vi "HeaderAction.vi"(0 "InstrClass":refnum<class "MultiHarp150.lvclass"> caption="DNL_LabVIEW Object in", 11 "error in (no error)":errorcluster caption="entrée d'erreur (pas d'erreur)") -> (4 "InstrClassOut":refnum<class "MultiHarp150.lvclass"> caption="DNL_LabVIEW Object out", 6 "DataNames":string[](array[string]), 8 "Instr Name":string, 10 "HeaderString":string, 13 "ArrDisplayNames":string[](array[string]), 14 "DisplayNames":string[](array[string]), 15 "error out":errorcluster caption="sortie d'erreur")   [LabVIEW 2019, in "MultiHarp150.lvclass"]
uses:
  MultiHarp150.lvclass
  C:/Programmes Labview/LabScanV1A/DevicesClass/BaseDevice/BaseDevice.lvclass
  <userlib>/MultiHarp150/MH_MeasMode.ctl
  <userlib>/MultiHarp150/MH_RefSource.ctl
  MultiHarp150.lvclass/MultiHarp150.ctl
  BaseDevice/BaseDevice.lvclass/BaseDevice.ctl
  BaseDevice/Accessor/GetBaseDataPath.vi
  BaseDevice/BaseDevice.lvclass
panel:
  out "refsource":T1
  out "Mode":T2 items=["HIST"=0, "T2"=2, "T3"=3]
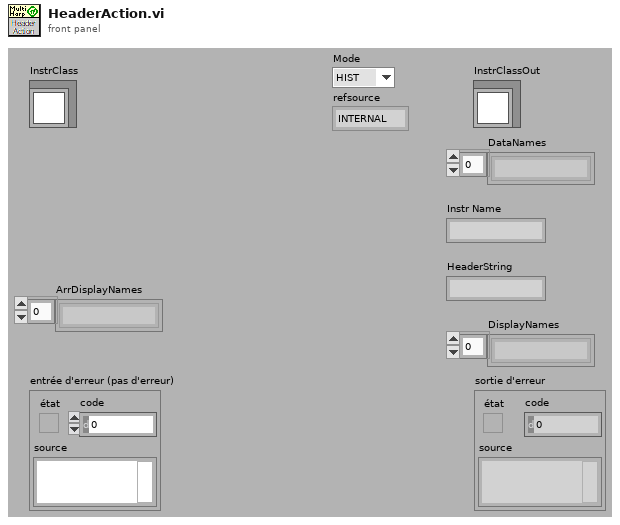
[diagram p1: front panel]
types:
  T1 = typedef "MH_RefSource.ctl" = enum16{"INTERNAL", "EXTERNAL_10MHZ", "WR_MASTER_GENERIC", "WR_SLAVE_GENERIC", "WR_GRANDM_GENERIC", "EXTN_GPS_PPS", "EXTN_GPS_PPS_UART", "WR_MASTER_MHARP", "WR_SLAVE_MHARP", "WR_GRANDM_MHARP"}
  T2 = typedef "MH_MeasMode.ctl" = i32
  T3 = typedef "MultiHarp150.lvclass/MultiHarp150_Func.ctl" = enum16{"ReadHistogram (Ph)", "ReadT2 (Ph)", "ReadT3 (Ph)", "ReadCount (Ph)"}
  T4 = typedef "MH_InputChannel_LS.ctl" = cluster{"Name":string, "Enable":bool, "Edge":i32, "Level":i32, "Offset":i32, "UseDeadTime":bool, "DeadTime":i32}
  T5 = cluster{"TagIdent":string, "TagIndex":i32, "TagType":i32, "TagValue":i64, "TagAuxData":string}[]
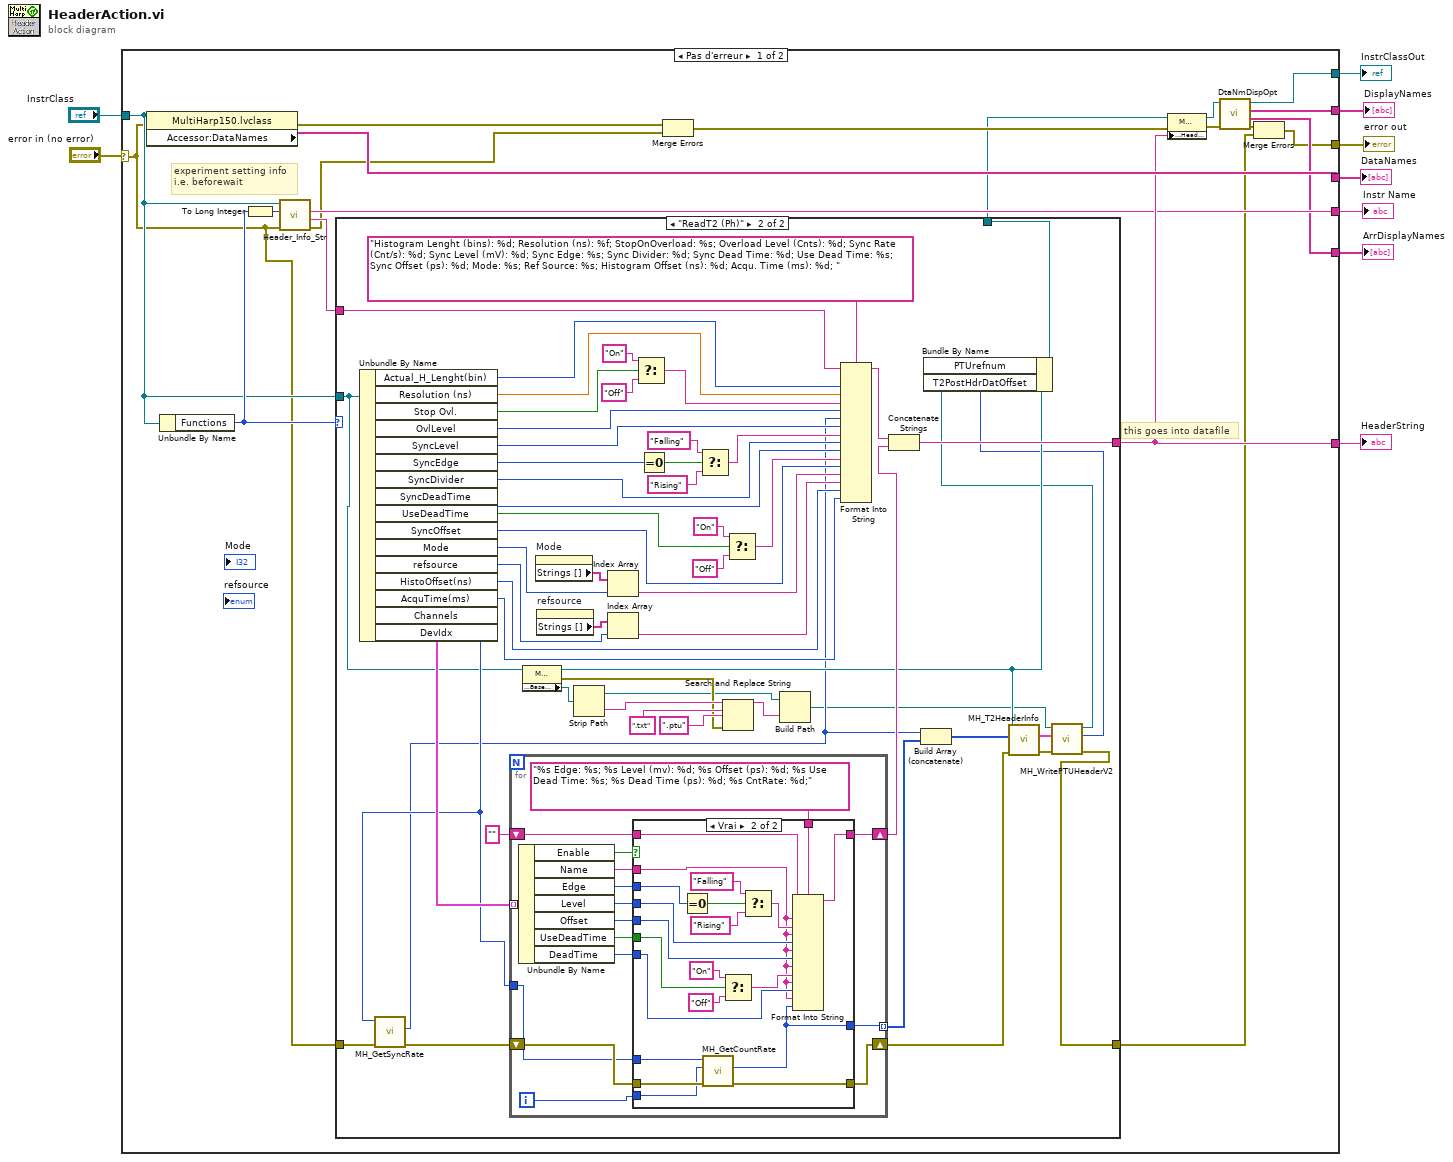
[diagram p0: block diagram]
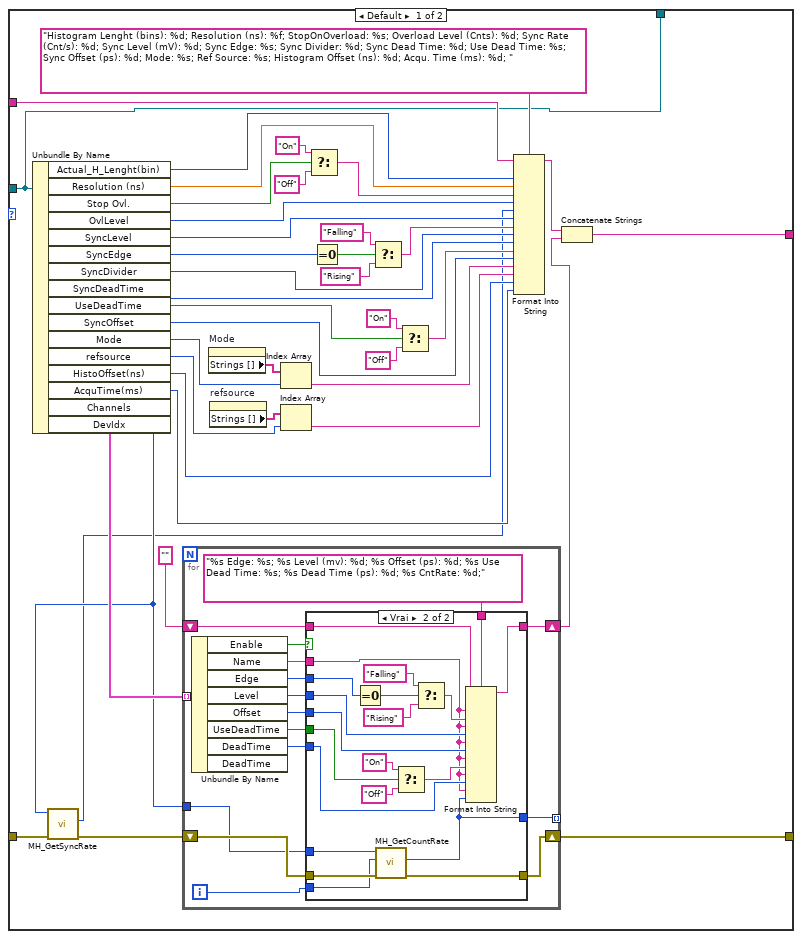
[diagram p2: hidden frame]
diagram:
  n1 = case shown="Pas d'erreur" "error in (no error)" {
    selector: "error in (no error)" -> [w14 w207]
    tunnel: [w27 _] -> w8
    tunnel: [w29 _] -> w7
    tunnel: "InstrClass" -> [w15 w208]
    tunnel: [w12 w207] -> w5
    tunnel: [w24 w208] -> w3
    tunnel: [w21 _] -> w4
    tunnel: [w22 _] -> w2
    tunnel: [w16 _] -> w1
    frame No Error {
      # "this goes into datafile"
      # "experiment setting info\ni.e. beforewait"
      n2 = property class="MultiHarp150.lvclass"(reference=w15, error in=w14) -> (error out=w28:errorcluster, "Accessor:DataNames"=w29:string[])  [unwired: 1 out]
      n3 = Unbundle By Name(w15) -> ("Functions"=w18:T3)
      n4 = To Long Integer(number=w18) -> (32bit integer=w17:i32)
      n5 = call-dynamic "Header_Info_Str.vi"("error in (no error)"=w14, "Functions"=w17, "DefaultDev in"=w15) -> ("error out"=w13:errorcluster, "HdrInfoStr"=w20:string, "InstrumentName"=w21:string)  [unwired: 5 in, 1 out]
      n6 = case shown="\"ReadT2 (Ph)\"" w18 {
        tunnel: [w39 w136] -> w27
        tunnel: w20 -> [w70 w167]
        tunnel: w15 -> [w30 w110]
        tunnel: w14 -> [w38 w135]
        tunnel: [w31 w124] -> w11
        tunnel: [w30 w113] -> w10
        frame Default {
          n7 = Unbundle By Name(w30) -> ("Actual_H_Lenght(bin)"=w48:i32, "Resolution (ns)"=w50:dbl, "Stop Ovl."=w52:bool, "OvlLevel"=w53:u32, "SyncLevel"=w34:i32, "SyncEdge"=w68:i32, "SyncDivider"=w64:i32, "SyncDeadTime"=w63:i32, "UseDeadTime"=w58:bool, "SyncOffset"=w49:i32, "Mode"=w55:T2, "refsource"=w44:T1, "HistoOffset(ns)"=w42:i32, "AcquTime(ms)"=w41:i32, "Channels"=w40:T4[], "DevIdx"=w36:i32)
          n8 = call <userlib>:"MH_GetSyncRate.vi"("error in (no error)"=w38, "devidx"=w36) -> ("error out"=w37:errorcluster, "syncrate"=w33:i32)  [unwired: 7 in, 1 out]
          n9 = for {
            tunnel: w40 -> [w86] mode=indexing
            shift-right: [w76] -> w32
            shift-left: "" -> [w77]
            tunnel: w36 -> [w74]
            shift-right: [w73] -> w31
            shift-left: w37 -> [w75]
            tunnel: [w71] -> _ mode=indexing
            i -> [w72]
            n10 = Unbundle By Name(w86) -> ("Enable"=w78:bool, "Name"=w79:string, "Edge"=w85:i32, "Level"=w82:i32, "Offset"=w81:i32, "UseDeadTime"=w84:bool, "DeadTime"=w80:i32)  [unwired: 1 out]
            n11 = case shown="Vrai" w78 {
              tunnel: w85 -> [_ w104]
              tunnel: w84 -> [_ w103]
              tunnel: "%s Edge: %s; %s Level (mv): %d; %s Offset (ps): %d; %s Use Dead Time: %s; %s Dead Time (ps): %d; %s CntRate: %d;" -> [_ w97]
              tunnel: w82 -> [_ w101]
              tunnel: w81 -> [_ w100]
              tunnel: w80 -> [_ w98]
              tunnel: w79 -> [_ w90]
              tunnel: w77 -> [w88 w96]
              tunnel: [w88 w95] -> w76
              tunnel: w75 -> [w87 w94]
              tunnel: w74 -> [_ w93]
              tunnel: [w87 w92] -> w73
              tunnel: w72 -> [_ w91]
              tunnel: [_ w89] -> w71
              frame False {
              }
              frame True {
                n12 = Equal To 0?(x=w104) -> (x = 0?=w106:bool)
                n13 = call <userlib>:"MH_GetCountRate.vi"("error in (no error)"=w94, "Channel"=w91, "devidx"=w93) -> ("error out"=w92:errorcluster, "rate"=w89:i32)  [unwired: 6 in, 1 out]
                n14 = Select(t="On", s=w103, f="Off") -> (s? t:f=w99:string)
                n15 = Select(t="Falling", s=w106, f="Rising") -> (s? t:f=w102:string)
                n16 = Format Into String(format string=w97, initial string=w96, w90, w102, w90, w101, w90, w100, w90, w99, w90, w98, w90, w89) -> (resulting string=w95:string)  [unwired: 1 in, 1 out]
              }
            }
          }
          n17 = property on="Mode" class="MDér (strict)"() -> ("Strings []"=w56:string[])  [unwired: 2 in, 2 out]
          n18 = property on="refsource" class="Énum (strict)"() -> ("Strings []"=w45:string[])  [unwired: 2 in, 2 out]
          n19 = Index Array(array=w56, index=w55) -> (element=w47:string)
          n20 = Index Array(array=w45, index=w44) -> (element=w43:string)
          n21 = Select(t="On", s=w52, f="Off") -> (s? t:f=w51:string)
          n22 = Equal To 0?(x=w68) -> (x = 0?=w67:bool)
          n23 = Select(t="Falling", s=w67, f="Rising") -> (s? t:f=w35:string)
          n24 = Select(t="On", s=w58, f="Off") -> (s? t:f=w57:string)
          n25 = Format Into String(format string="Histogram Lenght (bins): %d; Resolution (ns): %f; StopOnOverload: %s; Overload Level (Cnts): %d; Sync Rate (Cnt/s): %d; Sync Level (mV): %d; Sync Edge: %s; Sync Divider: %d; Sync Dead Time: %d; Use Dead Time: %s; Sync Offset (ps): %d; Mode: %s; Ref Source: %s; Histogram Offset (ns): %d; Acqu. Time (ms): %d; " ("chaîne de format"), initial string=w70, w48, w50, w51, w53, w33, w34, w35, w64, w63, w57, w49, w47, w43, w42, w41) -> (resulting string=w54:string)  [unwired: 1 in, 1 out]
          n26 = Concatenate Strings(w54, w32) -> (w39:string)
        }
        frame "ReadT2 (Ph)" {
          n27 = Unbundle By Name(w110) -> ("Actual_H_Lenght(bin)"=w145:i32, "Resolution (ns)"=w147:dbl, "Stop Ovl."=w149:bool, "OvlLevel"=w150:u32, "SyncLevel"=w131:i32, "SyncEdge"=w165:i32, "SyncDivider"=w161:i32, "SyncDeadTime"=w160:i32, "UseDeadTime"=w155:bool, "SyncOffset"=w146:i32, "Mode"=w152:T2, "refsource"=w141:T1, "HistoOffset(ns)"=w139:i32, "AcquTime(ms)"=w138:i32, "Channels"=w137:T4[], "DevIdx"=w133:i32)
          n28 = call <userlib>:"MH_GetSyncRate.vi"("error in (no error)"=w135, "devidx"=w133) -> ("error out"=w134:errorcluster, "syncrate"=w122:i32)  [unwired: 7 in, 1 out]
          n29 = for {
            tunnel: w137 -> [w183] mode=indexing
            shift-right: [w173] -> w130
            shift-left: "" -> [w174]
            tunnel: w133 -> [w171]
            shift-right: [w170] -> w127
            shift-left: w134 -> [w172]
            tunnel: [w168] -> w128 mode=indexing
            i -> [w169]
            n30 = Unbundle By Name(w183) -> ("Enable"=w175:bool, "Name"=w176:string, "Edge"=w182:i32, "Level"=w179:i32, "Offset"=w178:i32, "UseDeadTime"=w181:bool, "DeadTime"=w177:i32)
            n31 = case shown="Vrai" w175 {
              tunnel: w182 -> [_ w201]
              tunnel: w181 -> [_ w200]
              tunnel: "%s Edge: %s; %s Level (mv): %d; %s Offset (ps): %d; %s Use Dead Time: %s; %s Dead Time (ps): %d; %s CntRate: %d;" -> [_ w194]
              tunnel: w179 -> [_ w198]
              tunnel: w178 -> [_ w197]
              tunnel: w177 -> [_ w195]
              tunnel: w176 -> [_ w187]
              tunnel: w174 -> [w185 w193]
              tunnel: [w185 w192] -> w173
              tunnel: w172 -> [w184 w191]
              tunnel: w171 -> [_ w190]
              tunnel: [w184 w189] -> w170
              tunnel: w169 -> [_ w188]
              tunnel: [_ w186] -> w168
              frame False {
              }
              frame True {
                n32 = Equal To 0?(x=w201) -> (x = 0?=w203:bool)
                n33 = call <userlib>:"MH_GetCountRate.vi"("error in (no error)"=w191, "Channel"=w188, "devidx"=w190) -> ("error out"=w189:errorcluster, "rate"=w186:i32)  [unwired: 6 in, 1 out]
                n34 = Select(t="On", s=w200, f="Off") -> (s? t:f=w196:string)
                n35 = Select(t="Falling", s=w203, f="Rising") -> (s? t:f=w199:string)
                n36 = Format Into String(format string=w194, initial string=w193, w187, w199, w187, w198, w187, w197, w187, w196, w187, w195, w187, w186) -> (resulting string=w192:string)  [unwired: 1 in, 1 out]
              }
            }
          }
          n37 = property class="MultiHarp150.lvclass"(reference=w110) -> (reference out=w123:refnum<class "MultiHarp150.lvclass">, error out=w117:errorcluster, "Accessor:BaseDataPath"=w121:path)  [unwired: 1 in]
          n38 = property on="Mode" class="MDér (strict)"() -> ("Strings []"=w153:string[])  [unwired: 2 in, 2 out]
          n39 = property on="refsource" class="Énum (strict)"() -> ("Strings []"=w142:string[])  [unwired: 2 in, 2 out]
          n40 = Strip Path(path=w121) -> (stripped path=w116:path, name=w120:string)
          n41 = Index Array(array=w153, index=w152) -> (element=w144:string)
          n42 = Index Array(array=w142, index=w141) -> (element=w140:string)
          n43 = Select(t="On", s=w149, f="Off") -> (s? t:f=w148:string)
          n44 = Equal To 0?(x=w165) -> (x = 0?=w164:bool)
          n45 = Select(t="Falling", s=w164, f="Rising") -> (s? t:f=w132:string)
          n46 = Search and Replace String(input string=w120, search string=".txt" ("expression régulière"), replace string=".ptu" ("expression régulière"), error in=w117) -> (result string=w115:string)  [unwired: 4 in, 3 out]
          n47 = Select(t="On", s=w155, f="Off") -> (s? t:f=w154:string)
          n48 = Build Path(base path=w116, name or relative path=w115) -> (appended path=w114:path)
          n49 = Format Into String(format string="Histogram Lenght (bins): %d; Resolution (ns): %f; StopOnOverload: %s; Overload Level (Cnts): %d; Sync Rate (Cnt/s): %d; Sync Level (mV): %d; Sync Edge: %s; Sync Divider: %d; Sync Dead Time: %d; Use Dead Time: %s; Sync Offset (ps): %d; Mode: %s; Ref Source: %s; Histogram Offset (ns): %d; Acqu. Time (ms): %d; " ("chaîne de format"), initial string=w167, w145, w147, w148, w150, w122, w131, w132, w161, w160, w154, w146, w144, w140, w139, w138) -> (resulting string=w151:string)  [unwired: 1 in, 1 out]
          n50 = Concatenate Strings(w151, w130) -> (w136:string)
          n51 = Build Array (concatenate)(w122, w128) -> (w129:i32[])
          n52 = call "MH_T2HeaderInfo.vi"("entrée d'erreur"=w127, "CountRates"=w129, "InstrClass"=w123) -> ("sortie d'erreur"=w126:errorcluster, "HeaderTags"=w125:T5)  [unwired: 7 in]
          n53 = call <userlib>:"MH_WritePTUHeaderV2.vi"("entrée d'erreur"=w126, "TagArray"=w125, "Path"=w114) -> ("sortie d'erreur"=w124:errorcluster, "offset (in bytes)"=w111:i64, "refnum Out"=w112:refnum<file>)  [unwired: 6 in]
          n54 = Bundle By Name(cluster=w123, "PTUrefnum"=w112, "T2PostHdrDatOffset"=w111) -> (w113:refnum<class "MultiHarp150.lvclass">)
        }
      }
      n55 = Merge Errors(w28, w13) -> (w19:errorcluster)
      n56 = property class="MultiHarp150.lvclass"(reference=w10, error in=w19, "Accessor:HeaderString"=w27) -> (reference out=w23:refnum<class "MultiHarp150.lvclass">, error out=w26:errorcluster)
      n57 = call "DtaNmDispOpt.vi"("error in (no error)"=w26, "BaseDevice en entrée"=w23) -> ("error out"=w25:errorcluster, "ArrDisplayNames"=w16:string[], "DisplayNames"=w22:string[], "BaseDevice en sortie"=w24:refnum<class "MultiHarp150.lvclass">)  [unwired: 6 in]
      n58 = Merge Errors(w25, w11) -> (w12:errorcluster)
    }
    frame Error {
    }
  }
  "error out" <- w5
  "InstrClassOut" <- w3
  "DataNames" <- w7
  "HeaderString" <- w8
  "Instr Name" <- w4
  "DisplayNames" <- w2
  "ArrDisplayNames" <- w1
